vi "Set Keyboard Lighting.vi"(8 "error in (no error)":errorcluster, 11 "LED Color":u32(colorbox)) -> (0 "error out":errorcluster)   [LabVIEW 2022 SP3, in "Logitech Devices.lvlib"]
uses:
  Logitech Devices.lvlib
  C:/Program Files/LGHUB/sdks/sdk_legacy_led_x86.dll
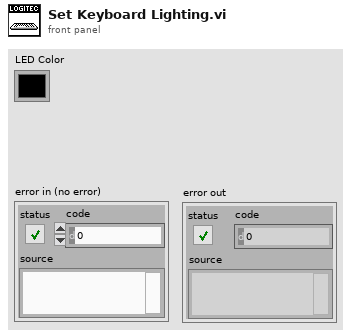
[diagram p1: front panel]
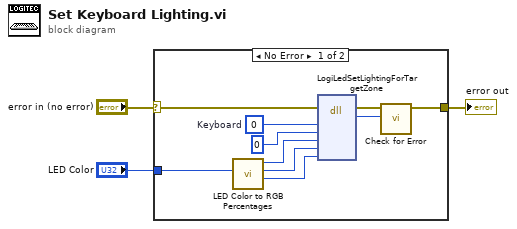
[diagram p0: block diagram]
diagram:
  n1 = case shown="No Error" "error in (no error)" {
    selector: "error in (no error)" -> [w13 w14]
    tunnel: [w6 w14] -> w2
    tunnel: "LED Color" -> [w11 _]
    frame No Error {
      w5 = u8 0  # Keyboard
      n2 = call "LED Color to RGB Percentages.vi"("LED Color"=w11) -> ("Blue %"=w8:u8, "Green %"=w9:u8, "Red %"=w10:u8)  [unwired: 8 in]
      n3 = dll-call lib="C:/Program Files/LGHUB/sdks/sdk_legacy_led_x86.dll" fn="LogiLedSetLightingForTargetZone"(error in=w13, "Device Type"=w5, "Zone"=u8 0, "Red Percentage"=w10, "Green Percentage"=w9, "Blue Percentage"=w8) -> (error out=w7:errorcluster, "return type"=w12:u8)  [unwired: 7 in, 1 out]
      n4 = call "Check for Error.vi"("DLL-call return value"=w12, "error in (no error)"=w7) -> ("error out"=w6:errorcluster)  [unwired: 9 in]
    }
    frame Error {
    }
  }
  "error out" <- w2
